vi "Open_script.vi"(8 "Script name":string="Script_1", 11 "Folder Path":path=path "R:/Programing/Scriping/home/lvuser/auto") -> (0 "error out":errorcluster, 3 "Byte Stream File out":refnum<file>)   [LabVIEW 2017, in "labview-standard-library.lvlib"]
uses:
  labview-standard-library.lvlib
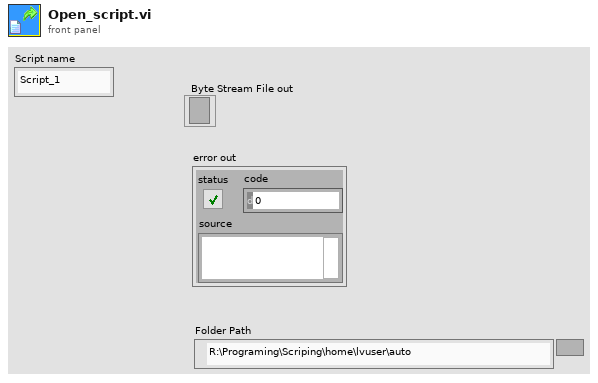
[diagram p1: front panel]
types:
  T1 = enum16{"open", "replace", "create", "open or create", "replace or create", "replace or create with confirmation"}
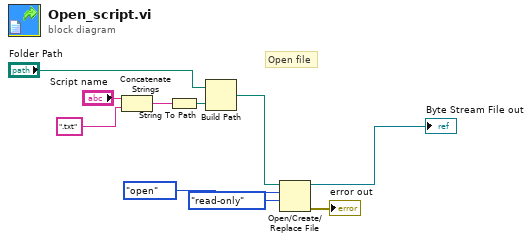
[diagram p0: block diagram]
diagram:
  # "Open file"
  n1 = Concatenate Strings("Script name", ".txt") -> (w2:string)
  n2 = String To Path(string=w2) -> (path=w7:path)
  n3 = Build Path(base path="Folder Path", name or relative path=w7) -> (appended path=w8:path)
  n4 = Open/Create/Replace File(file path (use dialog)=w8, operation (0:open)=T1."open", access (0:read/write)=enum16{"read/write", "read-only", "write-only"}."read-only") -> (refnum out=→"Byte Stream File out":refnum<file>, error out=→"error out":errorcluster)  [unwired: 3 in, 1 out]
